vi "Call Cypher Driver_genreal AFM.vi"(0 "Output Array":T1(array[cluster]), 1 "Offset":cluster{"X Offset":dbl, "Y Offset":dbl}, 3 "Move Z SetPoint":dbl, 5 "Distance Between Interpolated Points (nm)":dbl, 7 "Z Set Point (For Cypher AFM)":dbl, 9 "PID close":bool, 11 "Display the Wave (Cypher AFM)":bool, 12 "Image Size":cluster{"Width":dbl, "Height":dbl}) -> ()   [LabVIEW 2013]
doc: "This VI sends information in the correct format to the Cypher."
uses:
  simulator/Global Variables.vi
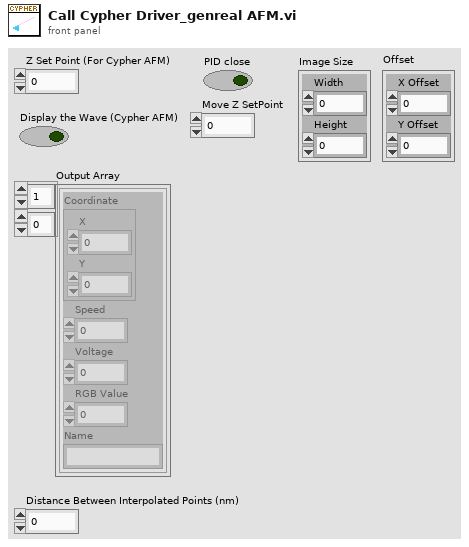
[diagram p1: front panel]
types:
  T1 = cluster{"Coordinate":cluster{"X":dbl, "Y":dbl}, "Speed":dbl, "Voltage":dbl, "RGB Value":i32, "Name":string}[][]
  T2 = cluster{"Coordinate":cluster{"X":dbl, "Y":dbl}, "Speed":dbl, "Voltage":dbl, "RGB Value":i32, "Name":string}
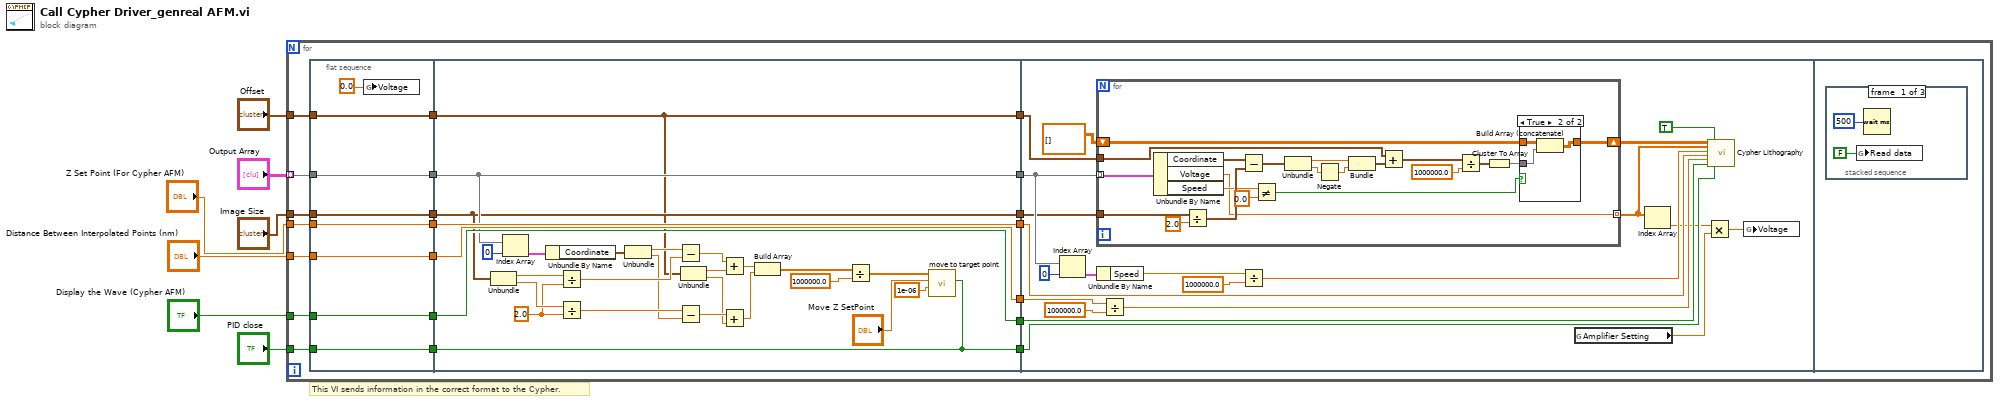
[diagram p0: block diagram]
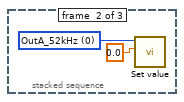
[diagram p3: hidden frame]
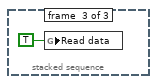
[diagram p4: hidden frame]
diagram:
  # "This VI sends information in the correct format to the Cypher."
  n1 = for {
    tunnel: "Distance Between Interpolated Points (nm)" -> [w23]
    tunnel: "Output Array" -> [w28] mode=indexing
    tunnel: "Z Set Point (For Cypher AFM)" -> [w27]
    tunnel: "Display the Wave (Cypher AFM)" -> [w26]
    tunnel: "PID close" -> [w25]
    tunnel: "Image Size" -> [w24]
    tunnel: "Offset" -> [w22]
    n2 = flat-sequence {
      tunnel: w22 -> [w30]
      tunnel: w23 -> [w31]
      tunnel: w24 -> [w32]
      tunnel: w25 -> [w33]
      tunnel: w26 -> [w34]
      tunnel: w27 -> [w35]
      tunnel: w28 -> [w36]
      tunnel: [w36] -> w14
      tunnel: [w35] -> w13
      tunnel: [w34] -> w12
      tunnel: [w33] -> w11
      tunnel: [w32] -> w10
      tunnel: [w31] -> w9
      tunnel: [w30] -> w8
      tunnel: [w40] -> w21
      tunnel: [w64] -> w20
      tunnel: [w63] -> w19
      tunnel: [w37] -> w18
      tunnel: [w39] -> w17
      tunnel: [w62] -> w16
      tunnel: [w38] -> w15
      tunnel: w14 -> [w40]
      tunnel: w13 -> [w64]
      tunnel: w12 -> [w63]
      tunnel: w11 -> [w37]
      tunnel: w10 -> [w39]
      tunnel: w9 -> [w62]
      tunnel: w8 -> [w38]
      tunnel: w21 -> [w85]
      tunnel: w20 -> [w81]
      tunnel: w19 -> [w80]
      tunnel: w18 -> [w79]
      tunnel: w17 -> [w78]
      tunnel: w16 -> [w73]
      tunnel: w15 -> [w69]
      frame #0 {
        n3 = global write "Global Variables.vi" "Voltage"(0.0 ("Voltage")) -> ()
      }
      frame #1 {
        w53 = 2.0 ("y")
        n4 = Unbundle(w39) -> ("Width"=w57:dbl, "Height"=w54:dbl)
        n5 = Index Array(array=w40, index=0 ("index (row)")) -> (element=w60:T2)
        n6 = Unbundle By Name(w60) -> ("Coordinate"=w58:cluster{"X":dbl, "Y":dbl})
        n7 = Divide(x=w57, y=w53) -> (x/y=w55:dbl)
        n8 = Divide(x=w54, y=w53) -> (x/y=w52:dbl)
        n9 = Unbundle(w58) -> ("X"=w56:dbl, "Y"=w51:dbl)
        n10 = Subtract(x=w56, y=w55) -> (x-y=w50:dbl)
        n11 = Subtract(x=w52, y=w51) -> (x-y=w48:dbl)
        n12 = Unbundle(w38) -> ("X Offset"=w49:dbl, "Y Offset"=w47:dbl)
        n13 = Add(x=w50, y=w49) -> (x+y=w46:dbl)
        n14 = Add(x=w48, y=w47) -> (x+y=w45:dbl)
        n15 = Build Array(w46, w45) -> (w43:dbl[])
        n16 = Divide(x=w43, y=1000000.0) -> (x/y=w42:dbl[])
        n17 = call "move to target point.vi"("PIS Close"=w37, "Litho Speed"=1e-06, "Z SetPoint"="Move Z SetPoint", "Target Point\n(  x      ,       y   )"=w42) -> ()  [unwired: 8 in]
      }
      frame #2 {
        n18 = Index Array(array=w85, index=0) -> (element=w83:T2)
        n19 = for {
          tunnel: w85 -> [w106] mode=indexing
          tunnel: [w86] -> w68 mode=indexing
          tunnel: w78 -> [w104]
          shift-right: [w94] -> w71
          shift-left: dbl[][] [] -> [w93]
          tunnel: w69 -> [w87]
          n20 = Unbundle By Name(w106) -> ("Coordinate"=w101:cluster{"X":dbl, "Y":dbl}, "Voltage"=w86:dbl, "Speed"=w92:dbl)
          n21 = Divide(x=w104, y=2.0) -> (x/y=w100:cluster{"Width":dbl, "Height":dbl})
          n22 = Subtract(x=w101, y=w100) -> (x-y=w99:cluster{dbl, dbl})
          n23 = Not Equal?(x=w92, y=0.0) -> (x != y?=w90:bool)
          n24 = Unbundle(w99) -> (w96:dbl, w98:dbl)
          n25 = Negate(x=w98) -> (-x=w97:dbl)
          n26 = Bundle(w96, w97) -> (w89:cluster{dbl, dbl})  [unwired: 1 in]
          n27 = Add(x=w87, y=w89) -> (x+y=w88:cluster{dbl, dbl})
          n28 = Divide(x=w88, y=1000000.0) -> (x/y=w102:cluster{dbl, dbl})
          n29 = Cluster To Array(cluster=w102) -> (array=w95:dbl[])
          n30 = case shown="True" w90 {
            tunnel: w95 -> [_ w110]
            tunnel: [w107 w109] -> w94
            tunnel: w93 -> [w107 w108]
            frame False {
            }
            frame True {
              n31 = Build Array (concatenate)(w108, w110) -> (w109:dbl[][])
            }
          }
        }
        n32 = Unbundle By Name(w83) -> ("Speed"=w76:dbl)
        n33 = Divide(x=w73, y=1000000.0) -> (x/y=w72:dbl)
        n34 = Divide(x=w76, y=1000000.0) -> (x/y=w75:dbl)
        n35 = global read "Global Variables.vi" "Amplifier Setting"() -> (w67:dbl)
        n36 = Index Array(array=w68) -> (element=w66:dbl)  [unwired: 1 in]
        n37 = Multiply(x=w66, y=w67) -> (x*y=w65:dbl)
        n38 = call "Cypher Lithography.vi"("Nodes on the line\n(  x      ,       y   )"=w71, "V"=w68, "Litho Speed"=w75, "Z SetPoint"=w81, "New nodes spacing"=w72, 5:w80, "Need interpolate new nodes?"=TRUE, "PID close"=w79) -> ()  [unwired: 12 in]
        n39 = global write "Global Variables.vi" "Voltage"(w65) -> ()
      }
      frame #3 {
        n40 = stacked-sequence {
          frame #0 {
            n41 = global write "Global Variables.vi" "Read data"(FALSE ("Read data")) -> ()
            n42 = Wait (ms)(milliseconds to wait=u32 500) -> ()  [unwired: 1 out]
          }
          frame #1 {
            w114 = u16 0 items=["OutA_52kHz", "OutB_52kHz", "OutC_78Hz", "PiezoX", "PiezoY", "PiezoZ", "DDS_Frequency1", "DDS_Frequency2", "DDS_Amplitude1", "DDS_Amplitude2", "DDS_DCOffset", "\"Setpoint%PIDSLoop.3\"", "\"Setpoint%PIDSLoop.4\"", ""] ("Output")
            n43 = call "Set value.vi"("Value"=0.0, "Output"=w114) -> ()  [unwired: 9 in, 1 out]
          }
          frame #2 {
            n44 = global write "Global Variables.vi" "Read data"(TRUE ("Read data")) -> ()
          }
        }
      }
    }
  }
